vi "ReadTunnel.vi"(1 "reference":refnum<vi>) -> (0 "Tunnel":T4)   [LabVIEW 2013]
uses:
  <vilib>/Utility/miscctls.llb/LVBoundsTypeDef.ctl
  <vilib>/Utility/miscctls.llb/LVPositionTypeDef.ctl
  <vilib>/Utility/miscctls.llb/LVRectTypeDef.ctl
panel:
  out "error out 16":errorcluster
  out "error out 15":errorcluster
  out "error out 14":errorcluster
  out "error out 13":errorcluster
  out "error out 12":errorcluster
  out "error out 11":errorcluster
  out "error out 10":errorcluster
  out "error out 9":errorcluster
  out "error out 8":errorcluster
  out "error out 7":errorcluster
  out "error out 6":errorcluster
  out "error out 5":errorcluster
  out "error out 4":errorcluster
  out "error out 3":errorcluster
  out "error out 2":errorcluster
  out "error out":errorcluster
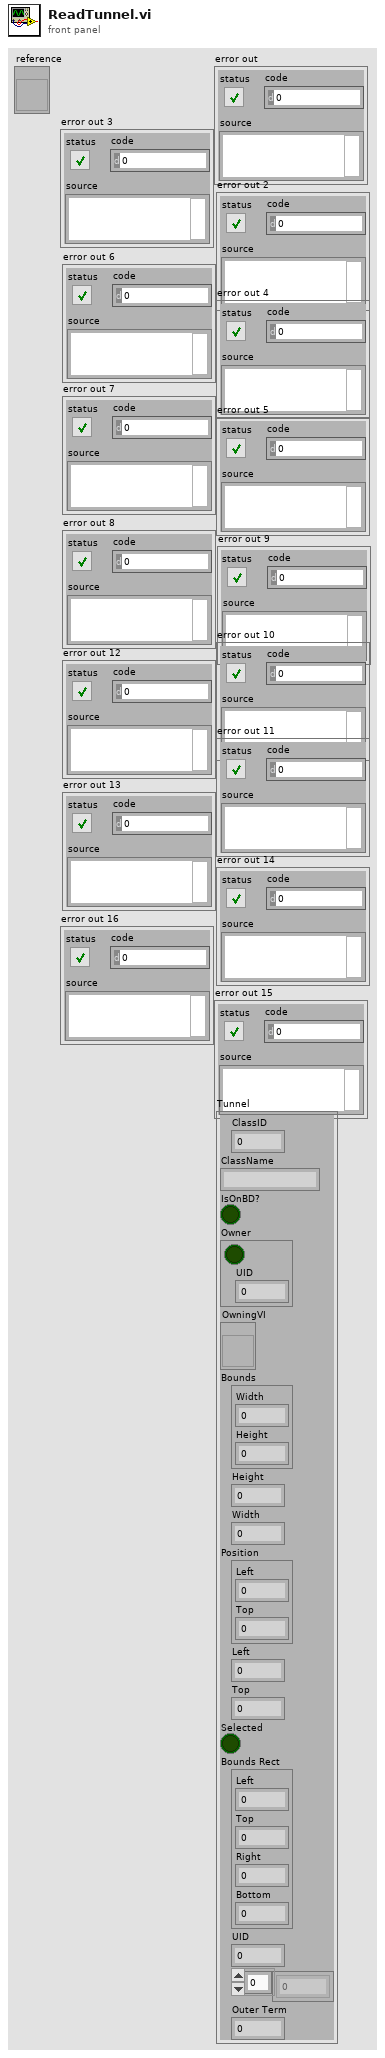
[diagram p1: front panel]
types:
  T1 = typedef "LVBoundsTypeDef.ctl" = cluster{"Width":u32, "Height":u32}
  T2 = typedef "LVPositionTypeDef.ctl" = cluster{"Left":i32, "Top":i32}
  T3 = typedef "LVRectTypeDef.ctl" = cluster{"Left":i16, "Top":i16, "Right":i16, "Bottom":i16}
  T4 = cluster{"ClassID":u32, "ClassName":string, "IsOnBD?":bool, "Owner":cluster{bool, "UID":i32}, "OwningVI":refnum<vi>, "Bounds":T1, "Height":u32, "Width":u32, "Position":T2, "Left":i32, "Top":i32, "Selected":bool, "Bounds Rect":T3, "UID":i32, "InsideTerms[]":i32[], "Outer Term":i32}
  T5 = cluster{"ClassID":u32, "ClassName":string, "IsOnBD?":bool, "Cluster":cluster{bool, "UID":i32}, "OwningVI":refnum<vi>, "Bounds":T1, "Height":u32, "Width":u32, "Position":T2, "Left":i32, "Top":i32, "Selected":bool, "Bounds Rect":T3, "UID":i32, i32[], "UID":i32}
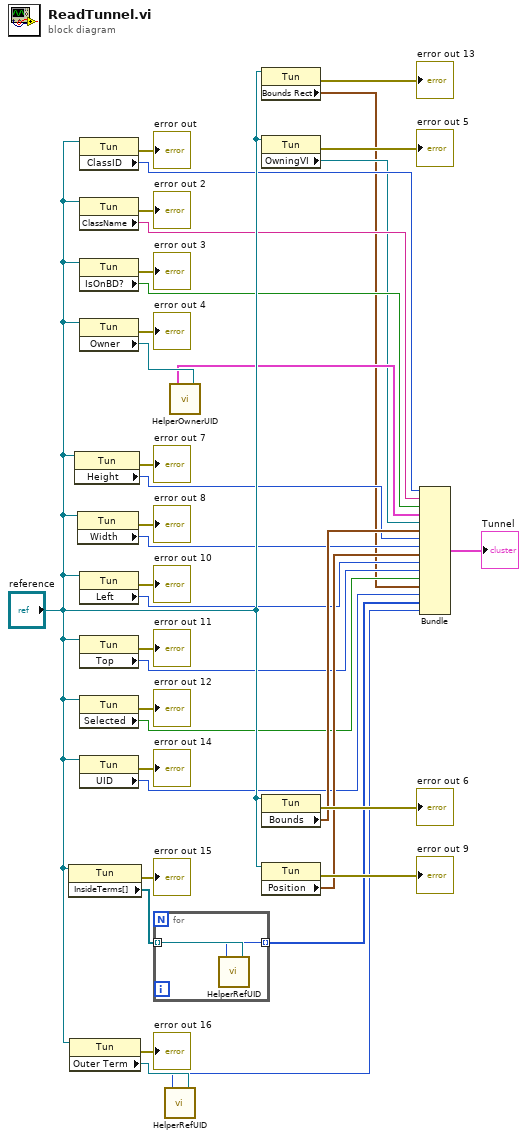
[diagram p0: block diagram]
diagram:
  n1 = property class="Tun"(reference="reference") -> (error out=→"error out 15":errorcluster, "InsideTerms[]"=w6:refnum<vi>[])  [unwired: 1 in, 1 out]
  n2 = property class="Tun"(reference="reference") -> (error out=→"error out 16":errorcluster, "Outer Term"=w3:refnum<vi>)  [unwired: 1 in, 1 out]
  n3 = property class="Tun"(reference="reference") -> (error out=→"error out 7":errorcluster, "Height"=w22:u32)  [unwired: 1 in, 1 out]
  n4 = property class="Tun"(reference="reference") -> (error out=→"error out 8":errorcluster, "Width"=w20:u32)  [unwired: 1 in, 1 out]
  n5 = property class="Tun"(reference="reference") -> (error out=→"error out":errorcluster, "ClassID"=w35:u32)  [unwired: 1 in, 1 out]
  n6 = property class="Tun"(reference="reference") -> (error out=→"error out 2":errorcluster, "ClassName"=w33:string)  [unwired: 1 in, 1 out]
  n7 = property class="Tun"(reference="reference") -> (error out=→"error out 3":errorcluster, "IsOnBD?"=w31:bool)  [unwired: 1 in, 1 out]
  n8 = property class="Tun"(reference="reference") -> (error out=→"error out 4":errorcluster, "Owner"=w29:refnum<vi>)  [unwired: 1 in, 1 out]
  n9 = property class="Tun"(reference="reference") -> (error out=→"error out 10":errorcluster, "Left"=w16:i32)  [unwired: 1 in, 1 out]
  n10 = property class="Tun"(reference="reference") -> (error out=→"error out 11":errorcluster, "Top"=w14:i32)  [unwired: 1 in, 1 out]
  n11 = property class="Tun"(reference="reference") -> (error out=→"error out 12":errorcluster, "Selected"=w12:bool)  [unwired: 1 in, 1 out]
  n12 = property class="Tun"(reference="reference") -> (error out=→"error out 14":errorcluster, "UID"=w8:i32)  [unwired: 1 in, 1 out]
  n13 = for {
    tunnel: w6 -> [w39] mode=indexing
    tunnel: [w38] -> w5 mode=indexing
    n14 = call "HelperRefUID.vi"("Text in"=w39) -> ("UID"=w38:i32)
  }
  n15 = call "HelperRefUID.vi"("Text in"=w3) -> ("UID"=w2:i32)
  n16 = call "HelperOwnerUID.vi"("Generic in"=w29) -> ("Cluster"=w28:cluster{bool, "UID":i32})
  n17 = property class="Tun"(reference="reference") -> (error out=→"error out 13":errorcluster, "Bounds Rect"=w10:T3)  [unwired: 1 in, 1 out]
  n18 = property class="Tun"(reference="reference") -> (error out=→"error out 5":errorcluster, "OwningVI"=w26:refnum<vi>)  [unwired: 1 in, 1 out]
  n19 = property class="Tun"(reference="reference") -> (error out=→"error out 6":errorcluster, "Bounds"=w24:T1)  [unwired: 1 in, 1 out]
  n20 = property class="Tun"(reference="reference") -> (error out=→"error out 9":errorcluster, "Position"=w18:T2)  [unwired: 1 in, 1 out]
  n21 = Bundle("ClassID"=w35, "ClassName"=w33, "IsOnBD?"=w31, "Cluster"=w28, "OwningVI"=w26, "Bounds"=w24, "Height"=w22, "Width"=w20, "Position"=w18, "Left"=w16, "Top"=w14, "Selected"=w12, "Bounds Rect"=w10, "UID"=w8, w5, "UID"=w2) -> (→"Tunnel":T5)  [unwired: 1 in]
